vi "C-885 Device Engine.vi"(0 "Unique Notifier Name":string, 11 "Axis Names":string[](array[string])) -> ()   [LabVIEW 2016]
uses:
  Stages Controls/Stage Actions.ctl
  Stages Controls/Stage Status.ctl
  Stages Controls/Stage Notifier Element.ctl
  C-885 Type Defs/C-885 Chassis Status.ctl
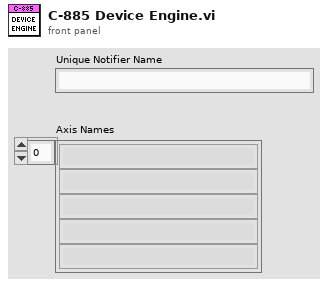
[diagram p1: front panel]
types:
  T1 = typedef "Stage Notifier Element.ctl" = cluster{"Action":T2, "Axis":bool[], "Setpoint":dbl[], "Velocity":dbl, "Cmd Recvd?":bool, "Position":dbl[], "Status":T3, "Misc":variant}
  T2 = typedef "Stage Actions.ctl" = enum16{"Get Position", "MVR", "MOVE", "HALT", "ONTARGET", "ERROR", "REFERENCE", "INIT", "VELOCITY", "STATUS", "EXIT", "HOME", "ZEROPOS", "NANOPOS", "ANALOG", "QUIT"}
  T3 = typedef "Stage Status.ctl" = enum16{"Error", "Abort", "Busy", "On Target"}
  T4 = typedef "C-885 Chassis Status.ctl" = enum16{"Avalible", "Busy", "Halt"}
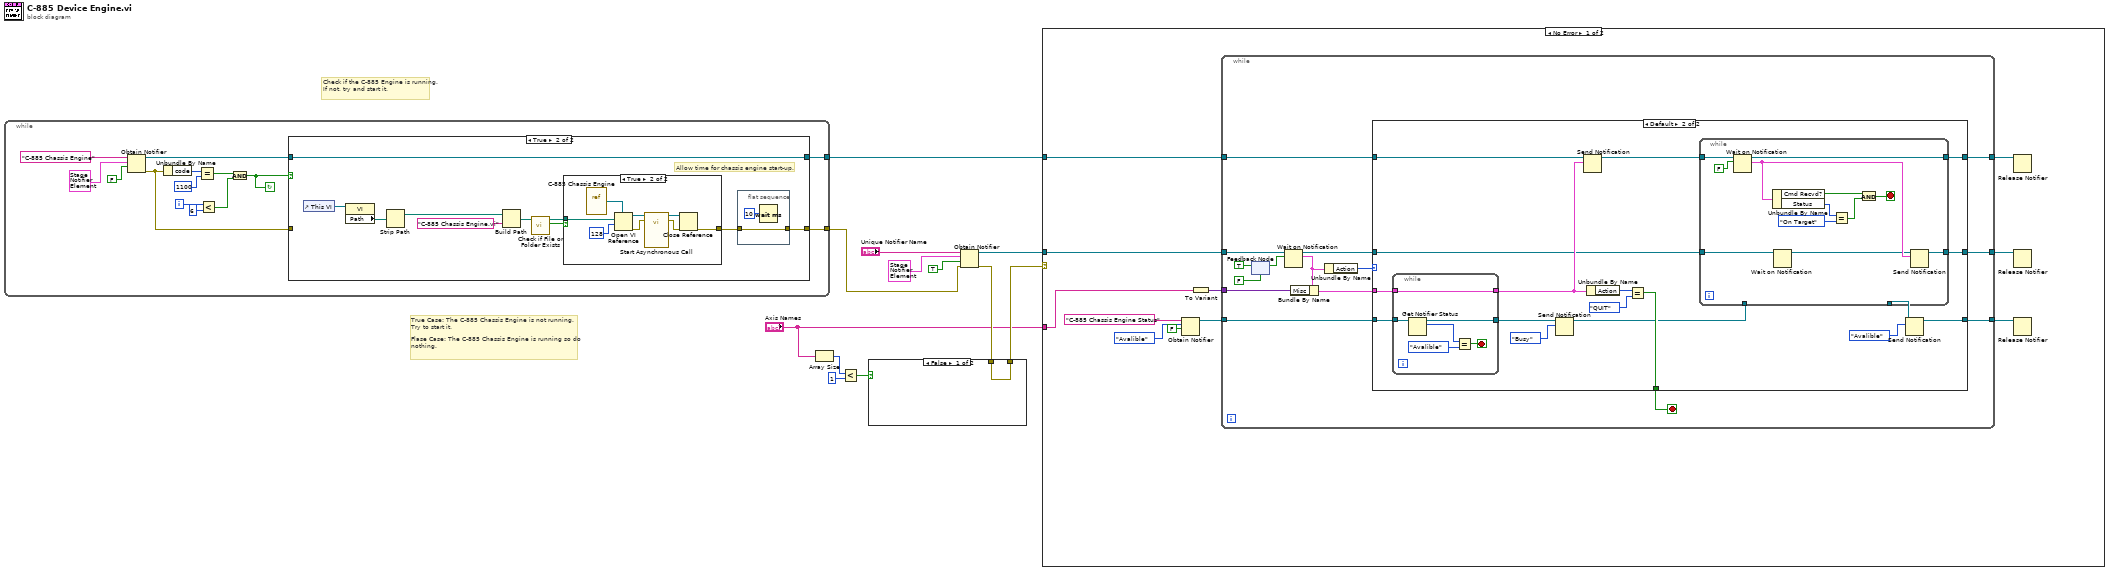
[diagram p0: block diagram]
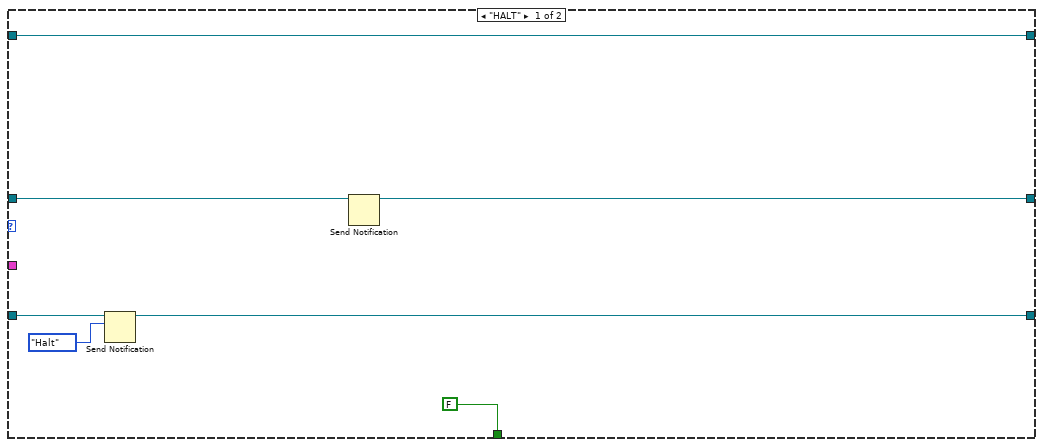
[diagram p2: hidden frame]
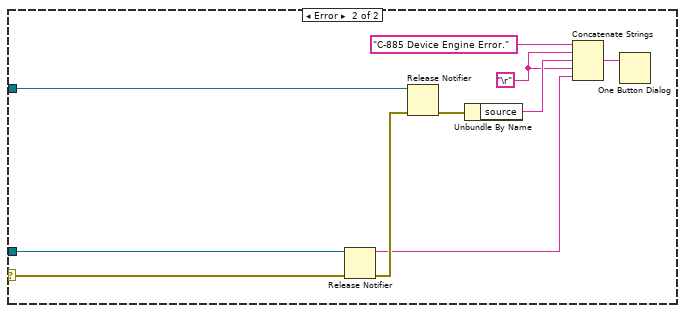
[diagram p3: hidden frame]
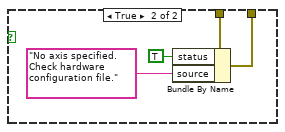
[diagram p4: hidden frame]
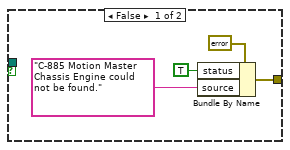
[diagram p6: hidden frame]
diagram:
  # "Check if the C-885 Engine is running. If not, try and start it."
  # "True Case: The C-885 Chassis Engine is not running.\nTry to start it.\n\nFlase Case: The C-885 Chassis Engine is running so do\nnothing."
  n1 = while {
    tunnel: [w20] -> w2
    tunnel: [w15] -> w9
    i -> [w22]
    stop <- w17 continue-if-true
    n2 = Obtain Notifier(name (unnamed)="C-885 Chassis Engine", notification data type=T1 {"Action"=enum."Get Position", "Axis"=[], "Setpoint"=[], "Velocity"=0.5, "Cmd Recvd?"=FALSE, "Position"=[], "Status"=enum."Error", "Misc"=variant} ("Stage Status"), create if not found? (T)=FALSE) -> (notifier out=w26:refnum<notifier>, error out=w14:errorcluster)  [unwired: 1 in, 1 out]
    n3 = Unbundle By Name(w14) -> ("code"=w25:i32)
    n4 = Equal?(x=w25, y=1100) -> (x = y?=w18:bool)
    n5 = Less?(x=w22, y=6) -> (x < y?=w19:bool)
    n6 = And(x=w18, y=w19) -> (x .and. y?=w17:bool)
    n7 = case shown="True" w17 {
      tunnel: w26 -> [w28 w38]
      tunnel: [w28 w38] -> w20
      tunnel: [w27 w29] -> w15
      tunnel: w14 -> [w27 _]
      frame False {
      }
      frame True {
        # "Allow time for chassis engine start-up."
        n8 = control-ref of="This VI"() -> (w33:refnum<vi>)
        n9 = property class="VI"(reference=w33) -> ("Path"=w34:path)  [unwired: 1 in, 2 out]
        n10 = Strip Path(path=w34) -> (stripped path=w35:path)  [unwired: 1 out]
        n11 = Build Path(base path=w35, name or relative path="C-885 Chassis Engine.vi" ("name (unnamed)")) -> (appended path=w37:path)
        n12 = call <vilib>:"Check if File or Folder Exists.vi"("path"=w37) -> ("file or folder exists?"=w32:bool, "dup path"=w31:path)  [unwired: 8 in, 1 out]
        n13 = case shown="True" w32 {
          tunnel: w31 -> [_ w46]
          tunnel: [w41 w45] -> w30
          frame False {
            n14 = Bundle By Name(cluster=errorcluster {"status"=FALSE, "code"=0, "source"=""} ("Error"), "status"=TRUE, "source"="C-885 Motion Master Chassis Engine could not be found.") -> (w41:errorcluster)
          }
          frame True {
            n15 = vi-ref "C-885 Chassis Engine.vi"() -> (w51:refnum<vi>)
            n16 = Open VI Reference(type specifier VI Refnum (for type only)=w51, vi path=w46, options=128) -> (vi reference=w50:refnum<vi>, error out=w48:errorcluster)  [unwired: 3 in]
            n17 = call-by-ref "Start Asynchronous Call"(reference=w50, error in=w48) -> (reference out=w49:refnum<vi>, error out=w47:errorcluster)  [unwired: 16 in]
            n18 = Close Reference(reference=w49, error in (no error)=w47) -> (error out=w45:errorcluster)
          }
        }
        n19 = flat-sequence {
          tunnel: w30 -> [w40]
          tunnel: [w40] -> w29
          frame #0 {
            n20 = Wait (ms)(milliseconds to wait=u32 10) -> ()  [unwired: 1 out]
          }
        }
      }
    }
  }
  n21 = Array Size(array="Axis Names") -> (size(s)=w8:i32)
  n22 = Less?(x=w8, y=1) -> (x < y?=w6:bool)
  n23 = Obtain Notifier(name (unnamed)="Unique Notifier Name", notification data type=T1 {"Action"=enum."INIT", "Axis"=[], "Setpoint"=[], "Velocity"=0.5, "Cmd Recvd?"=FALSE, "Position"=[], "Status"=enum."Error", "Misc"=variant} ("Stage Status"), create if not found? (T)=TRUE, error in (no error)=w9) -> (notifier out=w3:refnum<notifier>, error out=w5:errorcluster)  [unwired: 1 out]
  n24 = case shown="False" w6 {
    tunnel: w5 -> [w53 w57]
    tunnel: [w53 w54] -> w4
    frame False {
    }
    frame True {
      n25 = Bundle By Name(cluster=w57, "status"=TRUE, "source"="No axis specified. Check hardware configuration file.") -> (w54:errorcluster)
    }
  }
  n26 = case shown="No Error" w4 {
    selector: w4 -> [_ w133]
    tunnel: w3 -> [w68 w135]
    tunnel: w2 -> [w63 w134]
    tunnel: "Axis Names" -> [w67 _]
    frame No Error {
      n27 = Obtain Notifier(name (unnamed)="C-885 Chassis Engine Status", notification data type=C-885_Chassis_Status."Avalible" ("C-885 Status"), create if not found? (T)=FALSE) -> (notifier out=w59:refnum<notifier>)  [unwired: 1 in, 2 out]
      n28 = To Variant(anything=w67) -> (Variant=w66:variant)
      n29 = while {
        tunnel: w63 -> [w82]
        tunnel: w68 -> [w83]
        tunnel: w66 -> [w81]
        tunnel: [w78] -> w64
        tunnel: [w79] -> w65
        tunnel: w59 -> [w74]
        tunnel: [w71] -> w58
        stop <- w80 stop-if-true
        n30 = feedback #1(FALSE) -> (w75:bool)
        n31 = feedback-in #1(TRUE) -> ()
        n32 = Wait on Notification(notifier=w83, ignore previous (F)=w75) -> (notifier out=w72:refnum<notifier>, notification=w70:T1)  [unwired: 2 in, 2 out]
        n33 = Bundle By Name(cluster=w70, "Misc"=w81) -> (w73:T1)
        n34 = Unbundle By Name(w70) -> ("Action"=w69:T2)
        n35 = case shown="Default" w69 {
          tunnel: w82 -> [w86 w107]
          tunnel: [FALSE w104] -> w80
          tunnel: [w86 w102] -> w79
          tunnel: [w84 w101] -> w78
          tunnel: w74 -> [w88 w100]
          tunnel: w73 -> [_ w99]
          tunnel: w72 -> [w85 w95]
          tunnel: [w87 w91] -> w71
          frame "HALT" {
            n36 = Send Notification(notification=C-885_Chassis_Status."Halt", notifier=w88) -> (notifier out=w87:refnum<notifier>)  [unwired: 1 in, 1 out]
            n37 = Send Notification(notifier=w85) -> (notifier out=w84:refnum<notifier>)  [unwired: 2 in, 1 out]
          }
          frame Default {
            n38 = while {
              tunnel: w100 -> [w113]
              tunnel: [w109] -> w97
              tunnel: [w108] -> w98
              tunnel: w99 -> [w108]
              stop <- w110 stop-if-true
              n39 = Get Notifier Status(notifier=w113) -> (notifier out=w109:refnum<notifier>, current notification=w112:T4)  [unwired: 1 in, 3 out]
              n40 = Equal?(x=w112, y=C-885_Chassis_Status."Avalible") -> (x = y?=w110:bool)
            }
            n41 = Send Notification(notification=C-885_Chassis_Status."Busy", notifier=w97) -> (notifier out=w94:refnum<notifier>)  [unwired: 1 in, 1 out]
            n42 = Send Notification(notification=w98, notifier=w107) -> (notifier out=w103:refnum<notifier>)  [unwired: 1 in, 1 out]
            n43 = Unbundle By Name(w98) -> ("Action"=w106:T2)
            n44 = Equal?(x=w106, y=Stage_Actions."QUIT") -> (x = y?=w104:bool)
            n45 = while {
              tunnel: w103 -> [w125]
              tunnel: w95 -> [w115]
              tunnel: [w117] -> w102
              tunnel: [w116] -> w101
              tunnel: w94 -> [_]
              tunnel: [_] -> w93
              stop <- w118 stop-if-true
              n46 = Wait on Notification(notifier=w125, ignore previous (F)=FALSE) -> (notifier out=w117:refnum<notifier>, notification=w123:T1)  [unwired: 2 in, 2 out]
              n47 = Unbundle By Name(w123) -> ("Cmd Recvd?"=w120:bool, "Status"=w122:T3)
              n48 = Wait on Notification(notifier=w115) -> (notifier out=w114:refnum<notifier>)  [unwired: 3 in, 3 out]
              n49 = Equal?(x=w122, y=Stage_Status."On Target") -> (x = y?=w119:bool)
              n50 = And(x=w120, y=w119) -> (x .and. y?=w118:bool)
              n51 = Send Notification(notification=w123, notifier=w114) -> (notifier out=w116:refnum<notifier>)  [unwired: 1 in, 1 out]
            }
            n52 = Send Notification(notification=C-885_Chassis_Status."Avalible", notifier=w93) -> (notifier out=w91:refnum<notifier>)  [unwired: 1 in, 1 out]
          }
        }
      }
      n53 = Release Notifier(notifier=w65) -> ()  [unwired: 2 in, 3 out]
      n54 = Release Notifier(notifier=w64) -> ()  [unwired: 2 in, 3 out]
      n55 = Release Notifier(notifier=w58) -> ()  [unwired: 2 in, 3 out]
    }
    frame Error {
      w127 = "\r"
      n56 = Release Notifier(notifier=w135, error in (no error)=w133) -> (notifier name=w126:string, error out=w132:errorcluster)  [unwired: 1 in, 1 out]
      n57 = Release Notifier(notifier=w134, error in (no error)=w132) -> (error out=w128:errorcluster)  [unwired: 1 in, 2 out]
      n58 = Unbundle By Name(w128) -> ("source"=w130:string)
      n59 = Concatenate Strings("C-885 Device Engine Error.", w127, w130, w127, w126) -> (w129:string)
      n60 = One Button Dialog(message=w129) -> ()  [unwired: 1 in, 1 out]
    }
  }
